vi "Extract Data.vi"(8 "error in (no error)":errorcluster caption="entrée d'erreur (pas d'erreur)", 11 "Parsing Data RADIO_ERP1 en entrée":refnum<class "Parsing Data RADIO_ERP1_A5_H.lvclass">) -> (0 "error out":errorcluster caption="sortie d'erreur", 3 "Parsing Data RADIO_ERP1 en sortie":refnum<class "Parsing Data RADIO_ERP1_A5_H.lvclass">)   [LabVIEW 2020, in "Library Instrument & Equipement.lvlib" / "Library UART.lvlib" / "Parsing Data RADIO_ERP1_A5_H.lvclass"]
uses:
  Parsing Data RADIO_ERP1_A5_H.lvclass
  C:/Users/ngarcin/OneDrive - Altyor/Standard TB/Class/UART/UART Enocean/Parsing Data Enocean (Default)/Parsing Data Enocean (Default).lvclass
  Parsing Data RADIO_ERP1_A5_H.lvclass/Parsing Data RADIO_ERP1_A5_H.ctl
  Commun VI/Library Commun.lvlib
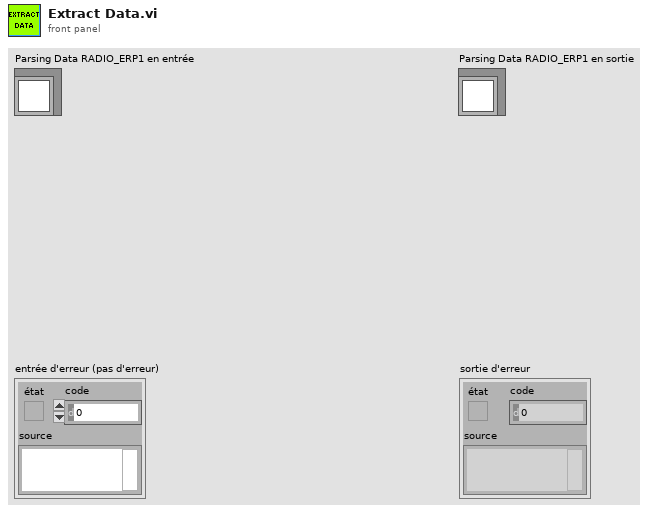
[diagram p1: front panel]
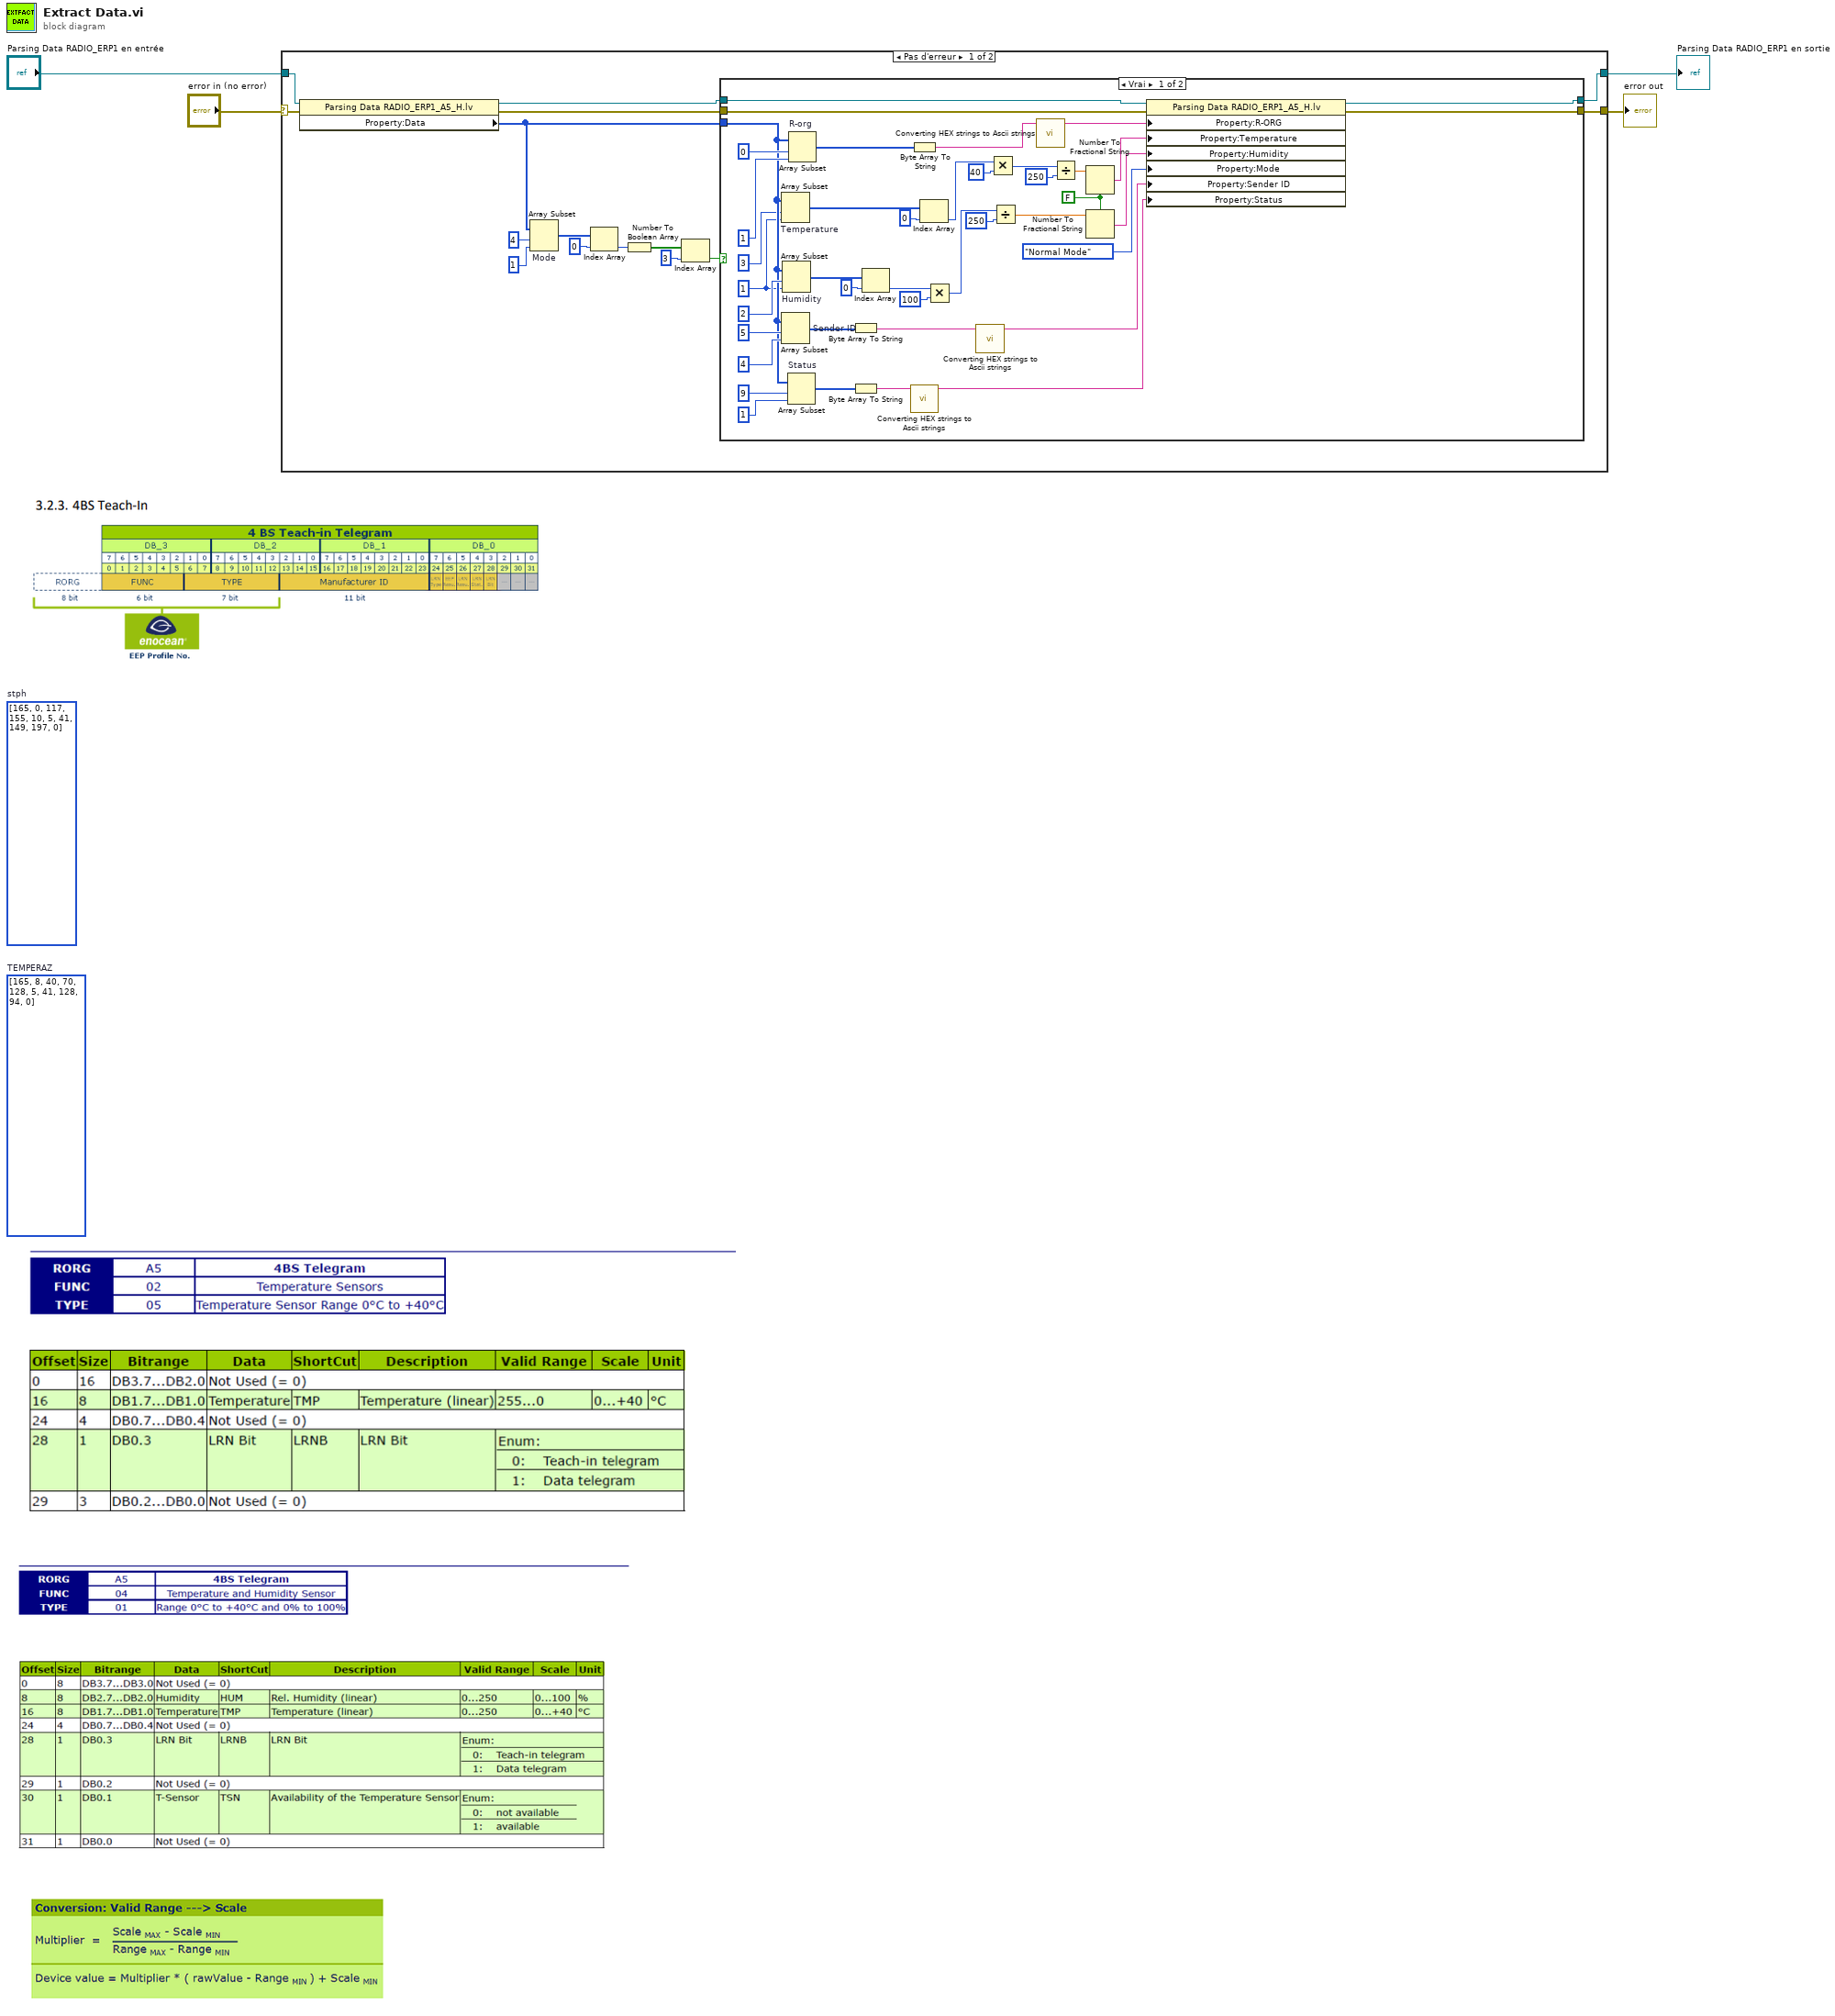
[diagram p0: block diagram]
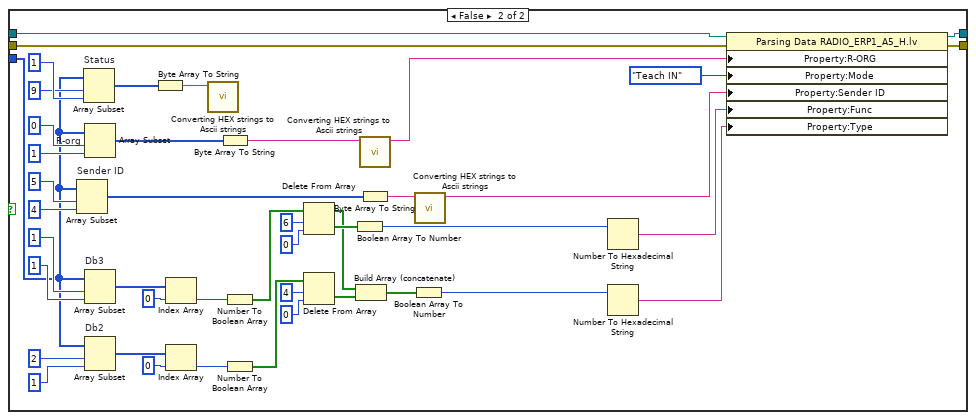
[diagram p2: hidden frame]
diagram:
  (unwired) u8[] [165, 0, 117, 155, 10, 5, 41, 149, 197, 0]  # stph
  (unwired) u8[] [165, 8, 40, 70, 128, 5, 41, 128, 94, 0]  # TEMPERAZ
  n1 = case shown="Pas d'erreur" "error in (no error)" {
    selector: "error in (no error)" -> [w15 w106]
    tunnel: [w14 w106] -> w3
    tunnel: [w16 w105] -> w1
    tunnel: "Parsing Data RADIO_ERP1 en entrée" -> [w17 w105]
    frame No Error {
      n2 = property class="Parsing Data RADIO_ERP1_A5_H.lv"(reference=w17, error in=w15) -> (reference out=w19:refnum<class "Parsing Data RADIO_ERP1_A5_H.lvclass">, error out=w18:errorcluster, "Property:Data"=w6:u8[])
      n3 = Array Subset "Mode"(array=w6, index=4 ("indice"), length=1 ("longueur")) -> (w11:u8[])
      n4 = Index Array(array=w11, index=0 ("indice")) -> (element=w7:u8)
      n5 = Number To Boolean Array(number=w7) -> (Boolean array=w9:bool[])
      n6 = Index Array(array=w9, index=3 ("indice")) -> (element=w5:bool)
      n7 = case shown="Vrai" w5 {
        tunnel: w19 -> [w60 w104]
        tunnel: w18 -> [w49 w94]
        tunnel: [w48 w93] -> w16
        tunnel: [w47 w92] -> w14
        tunnel: w6 -> [w35 w72]
        frame True {
          w20 = FALSE ("utiliser le séparateur décimal du système (V)")
          w34 = 1 ("longueur")
          n8 = Array Subset "Temperature"(array=w35, index=3 ("indice"), length=w34) -> (w31:u8[])
          n9 = Array Subset "Sender ID"(array=w35, index=5 ("indice"), length=4 ("longueur")) -> (w55:u8[])
          n10 = Array Subset "Humidity"(array=w35, index=2 ("indice"), length=w34) -> (w40:u8[])
          n11 = Array Subset "Status"(array=w35, index=9 ("indice"), length=1 ("indice")) -> (w50:u8[])
          n12 = Array Subset "R-org"(array=w35, index=0 ("indice"), length=1 ("longueur")) -> (w58:u8[])
          n13 = Byte Array To String(unsigned byte array=w55) -> (string=w54:string)
          n14 = Byte Array To String(unsigned byte array=w50) -> (string=w52:string)
          n15 = Index Array(array=w40, index=0 ("indice")) -> (element=w23:u8)
          n16 = Byte Array To String(unsigned byte array=w58) -> (string=w57:string)
          n17 = call "Converting HEX strings to Ascii strings.vi"("chaîne IN"=w52) -> ("Chaîne OUT"=w51:string)  [unwired: 9 in, 1 out]
          n18 = Index Array(array=w31, index=0 ("indice")) -> (element=w30:u8)
          n19 = Multiply(x=w23, y=u16 100 ("x")) -> (x*y=w26:u16)
          n20 = call "Converting HEX strings to Ascii strings.vi"("chaîne IN"=w54) -> ("Chaîne OUT"=w53:string)  [unwired: 9 in, 1 out]
          n21 = Multiply(x=w30, y=u16 40 ("x")) -> (x*y=w28:u16)
          n22 = Divide(x=w26, y=u16 250) -> (x/y=w22:dbl)
          n23 = call "Converting HEX strings to Ascii strings.vi"("chaîne IN"=w57) -> ("Chaîne OUT"=w56:string)  [unwired: 9 in, 1 out]
          n24 = Divide(x=w28, y=u16 250) -> (x/y=w27:dbl)
          n25 = Number To Fractional String(use system decimal point (T)=w20, number=w27) -> (F-format string=w39:string)  [unwired: 2 in]
          n26 = Number To Fractional String(use system decimal point (T)=w20, number=w22) -> (F-format string=w21:string)  [unwired: 2 in]
          n27 = property class="Parsing Data RADIO_ERP1_A5_H.lv"(reference=w60, error in=w49, "Property:R-ORG"=w56, "Property:Temperature"=w39, "Property:Humidity"=w21, "Property:Mode"=enum16{"Teach IN", "Normal Mode"}."Normal Mode" ("Mode"), "Property:Sender ID"=w53, "Property:Status"=w51) -> (reference out=w48:refnum<class "Parsing Data RADIO_ERP1_A5_H.lvclass">, error out=w47:errorcluster)
        }
        frame False {
          n28 = Array Subset "Sender ID"(array=w72, index=5 ("indice"), length=4 ("longueur")) -> (w99:u8[])
          n29 = Array Subset "Status"(array=w72, index=9 ("indice"), length=1 ("indice")) -> (w95:u8[])
          n30 = Array Subset "R-org"(array=w72, index=0 ("indice"), length=1 ("longueur")) -> (w102:u8[])
          n31 = Array Subset "Db3"(array=w72, index=1 ("indice"), length=1 ("longueur")) -> (w83:u8[])
          n32 = Array Subset "Db2"(array=w72, index=2 ("indice"), length=1 ("longueur")) -> (w71:u8[])
          n33 = Byte Array To String(unsigned byte array=w95) -> (string=w96:string)
          n34 = Index Array(array=w83, index=0 ("indice")) -> (element=w81:u8)
          n35 = Index Array(array=w71, index=0 ("indice")) -> (element=w70:u8)
          n36 = call "Converting HEX strings to Ascii strings.vi"("chaîne IN"=w96) -> ()  [unwired: 9 in, 2 out]
          n37 = Byte Array To String(unsigned byte array=w102) -> (string=w101:string)
          n38 = Number To Boolean Array(number=w81) -> (Boolean array=w80:bool[])
          n39 = Number To Boolean Array(number=w70) -> (Boolean array=w69:bool[])
          n40 = Delete From Array(array=w80, length=6 ("longueur"), index=0 ("indice")) -> (deleted portion=w78:bool[], array with subset deleted=w67:bool[])
          n41 = Delete From Array(array=w69, length=4 ("longueur"), index=0 ("indice")) -> (deleted portion=w66:bool[])  [unwired: 1 out]
          n42 = Boolean Array To Number(Boolean array=w78) -> (number=w77:u32)
          n43 = Build Array (concatenate)(w67, w66) -> (w64:bool[])
          n44 = call "Converting HEX strings to Ascii strings.vi"("chaîne IN"=w101) -> ("Chaîne OUT"=w100:string)  [unwired: 9 in, 1 out]
          n45 = Byte Array To String(unsigned byte array=w99) -> (string=w98:string)
          n46 = Boolean Array To Number(Boolean array=w64) -> (number=w65:u32)
          n47 = call "Converting HEX strings to Ascii strings.vi"("chaîne IN"=w98) -> ("Chaîne OUT"=w97:string)  [unwired: 9 in, 1 out]
          n48 = Number To Hexadecimal String(2:w77) -> (0:w76:string)  [unwired: 1 in]
          n49 = Number To Hexadecimal String(2:w65) -> (0:w63:string)  [unwired: 1 in]
          n50 = property class="Parsing Data RADIO_ERP1_A5_H.lv"(reference=w104, error in=w94, "Property:R-ORG"=w100, "Property:Mode"=enum16{"Teach IN", "Normal Mode"}."Teach IN" ("Mode"), "Property:Sender ID"=w97, "Property:Func"=w76, "Property:Type"=w63) -> (reference out=w93:refnum<class "Parsing Data RADIO_ERP1_A5_H.lvclass">, error out=w92:errorcluster)
        }
      }
    }
    frame Error {
    }
  }
  "error out" <- w3
  "Parsing Data RADIO_ERP1 en sortie" <- w1
